vi "Process_Event.vi"(8 "Status/Errors in":refnum<vi>, 9 "Control Parameters [] in":T16[](array[typedef]) {"Aux Byte Value" format="%02x"; "Max Real Value" format="%#_6e"; "Min Real Value" format="%#_6e"; "dReal/dByte" format="%#_6e"; "Byte Value" format="%02x"; "Identifier" format="%02x"}, 10 "Main parameters in":T1={"Mode"={"Mode"=enum."Dialog", "Expert?"=FALSE, "Dialog?"=FALSE}, "Stop loop"={"Settings changed?"=FALSE, "Stop?"=refnum}, "Send message"={"Send mode"=enum."Get parameters", "Set parameter list"=0, "Get parameter list"=0, "Reset device"=0, "Length set settings message"=0, "Reset buttons?"=FALSE, "Reset Master?"=enum."General"}, "Write settings"={"Options"=enum."File 1"}, "Settings state"={"MAS locked?"=refnum, "SLV locked?"=refnum}, "Button refs"={"Stop program"=refnum, "Save settings"=refnum, "DAQ mode"=refnum, "Reset settings"=refnum, "Apply settings"=refnum, "Reset MAS"=refnum, "Reset SLV"=refnum, "Local DBase?"=refnum, "Last value DBase"=FALSE, "Database"=refnum, "Calibration"=refnum, "Save settings 2"=refnum}, "Update screen"={"Detector number"=0, "Hardware"=enum."None"}, "Files"={"Path config file"=path "", "Path def. ini file"=path "", "Path ini file 1"=path "", "Path ini file 2"=path "", "Path RBF file"=path ""}, "DB connection"={"connection reference"=refnum, "Connected?"=refnum, "ODBC Name"=""}, "Status_id"=refnum, "Time difference"=refnum, "Satellites"=refnum, "Alignment parameters"=refnum, "Page Statistics 2"=refnum, "Database"=refnum, "Page Statistics"=refnum} {"Update screen"."Detector number" format="%#.0f"; "Send message"."Reset device" format="%x"; "Send message"."Get parameter list" format="%x"; "Send message"."Set parameter list" format="%x"}, 11 "Event array":u8[](array[numeric])) -> (0 "Status/Errors out":refnum<vi>, 1 "Main parameters out":T1={"Mode"={"Mode"=enum."Dialog", "Expert?"=FALSE, "Dialog?"=FALSE}, "Stop loop"={"Settings changed?"=FALSE, "Stop?"=refnum}, "Send message"={"Send mode"=enum."Get parameters", "Set parameter list"=0, "Get parameter list"=0, "Reset device"=0, "Length set settings message"=0, "Reset buttons?"=FALSE, "Reset Master?"=enum."General"}, "Write settings"={"Options"=enum."File 1"}, "Settings state"={"MAS locked?"=refnum, "SLV locked?"=refnum}, "Button refs"={"Stop program"=refnum, "Save settings"=refnum, "DAQ mode"=refnum, "Reset settings"=refnum, "Apply settings"=refnum, "Reset MAS"=refnum, "Reset SLV"=refnum, "Local DBase?"=refnum, "Last value DBase"=FALSE, "Database"=refnum, "Calibration"=refnum, "Save settings 2"=refnum}, "Update screen"={"Detector number"=0, "Hardware"=enum."None"}, "Files"={"Path config file"=path "", "Path def. ini file"=path "", "Path ini file 1"=path "", "Path ini file 2"=path "", "Path RBF file"=path ""}, "DB connection"={"connection reference"=refnum, "Connected?"=refnum, "ODBC Name"=""}, "Status_id"=refnum, "Time difference"=refnum, "Satellites"=refnum, "Alignment parameters"=refnum, "Page Statistics 2"=refnum, "Database"=refnum, "Page Statistics"=refnum} {"Update screen"."Detector number" format="%#.0f"; "Send message"."Reset device" format="%x"; "Send message"."Get parameter list" format="%x"; "Send message"."Set parameter list" format="%x"}, 2 "Event statistics":T15[](array[typedef]), 3 "Event cluster":T17={"Det_Numb"=0, "GPS_Timestamp"="", "Trigger_Pattern"={"Master ch. 1 lower threshold"=FALSE, "Master ch. 1 higher threshold"=FALSE, "Master ch. 2 lower threshold"=FALSE, "Master ch. 2 higher threshold"=FALSE, "Slave ch. 1 lower threshold"=FALSE, "Slave ch. 1 higher threshold"=FALSE, "Slave ch. 2 lower threshold"=FALSE, "Slave ch. 2 higher threshold"=FALSE, "External trigger"=FALSE, "Slave present?"=FALSE, "Ch. 1 low comparator master"=FALSE, "Ch. 1 high comparator master"=FALSE, "Ch. 2 low comparator master"=FALSE, "Ch. 2 high comparator master"=FALSE, "Ch. 1 low comparator slave"=FALSE, "Ch. 1 high comparator slave"=FALSE, "Ch. 2 low comparator slave"=FALSE, "Ch. 2 high comparator slave"=FALSE}, "Traces"=[], "MAS_Status_Events"=FALSE, "MAS_Vers_Numb"="Hardware: 0    FPGA: 0", "SLV_Status_Events"=FALSE, "SLV_Vers_Numb"="Hardware: 0    FPGA: 0", "DBase_connected?"=FALSE, "MAS_GPS_Long"=0.0, "MAS_GPS_Lat"=0.0, "MAS_GPS_Alt"=0.0, "Hardware"=enum."None"} {"MAS_GPS_Alt" format="%.2g"; "MAS_GPS_Lat" format="%#.7f"; "MAS_GPS_Long" format="%#.7f"})   [LabVIEW 2013]
uses:
  Controls/TabPage_Events.ctl
  Controls/Control_Parameters.ctl
  Controls/Master.ctl
  Controls/Event_Statistics.ctl
  Controls/Main_Parameters.ctl
  Controls/Mode.ctl
  Controls/Stop_Loop.ctl
  Controls/Send_Message.ctl
  Controls/Send_Message_Mode.ctl
  Controls/Write_Settings.ctl
  Controls/Write_Settings_Options.ctl
  Controls/Settings_State.ctl
  Controls/Button_Refs.ctl
  Controls/Update_Screen.ctl
  Controls/Files.ctl
  Controls/DB_Connection.ctl
  database/Connection.llb/Conn ObjectReference.ctl
  Controls/Get_Set_Statistics_Options2.ctl
panel:
  in  "Start counting?":bool=TRUE
  out "timer":u32
  in  "Start counting":bool=TRUE
  out "timer":u32
  out "Last trace":dbl[][](array[numeric])
  out "Show traces? 2":bool
  out "Show traces?":bool
  out "Last trace":dbl[][](array[numeric])
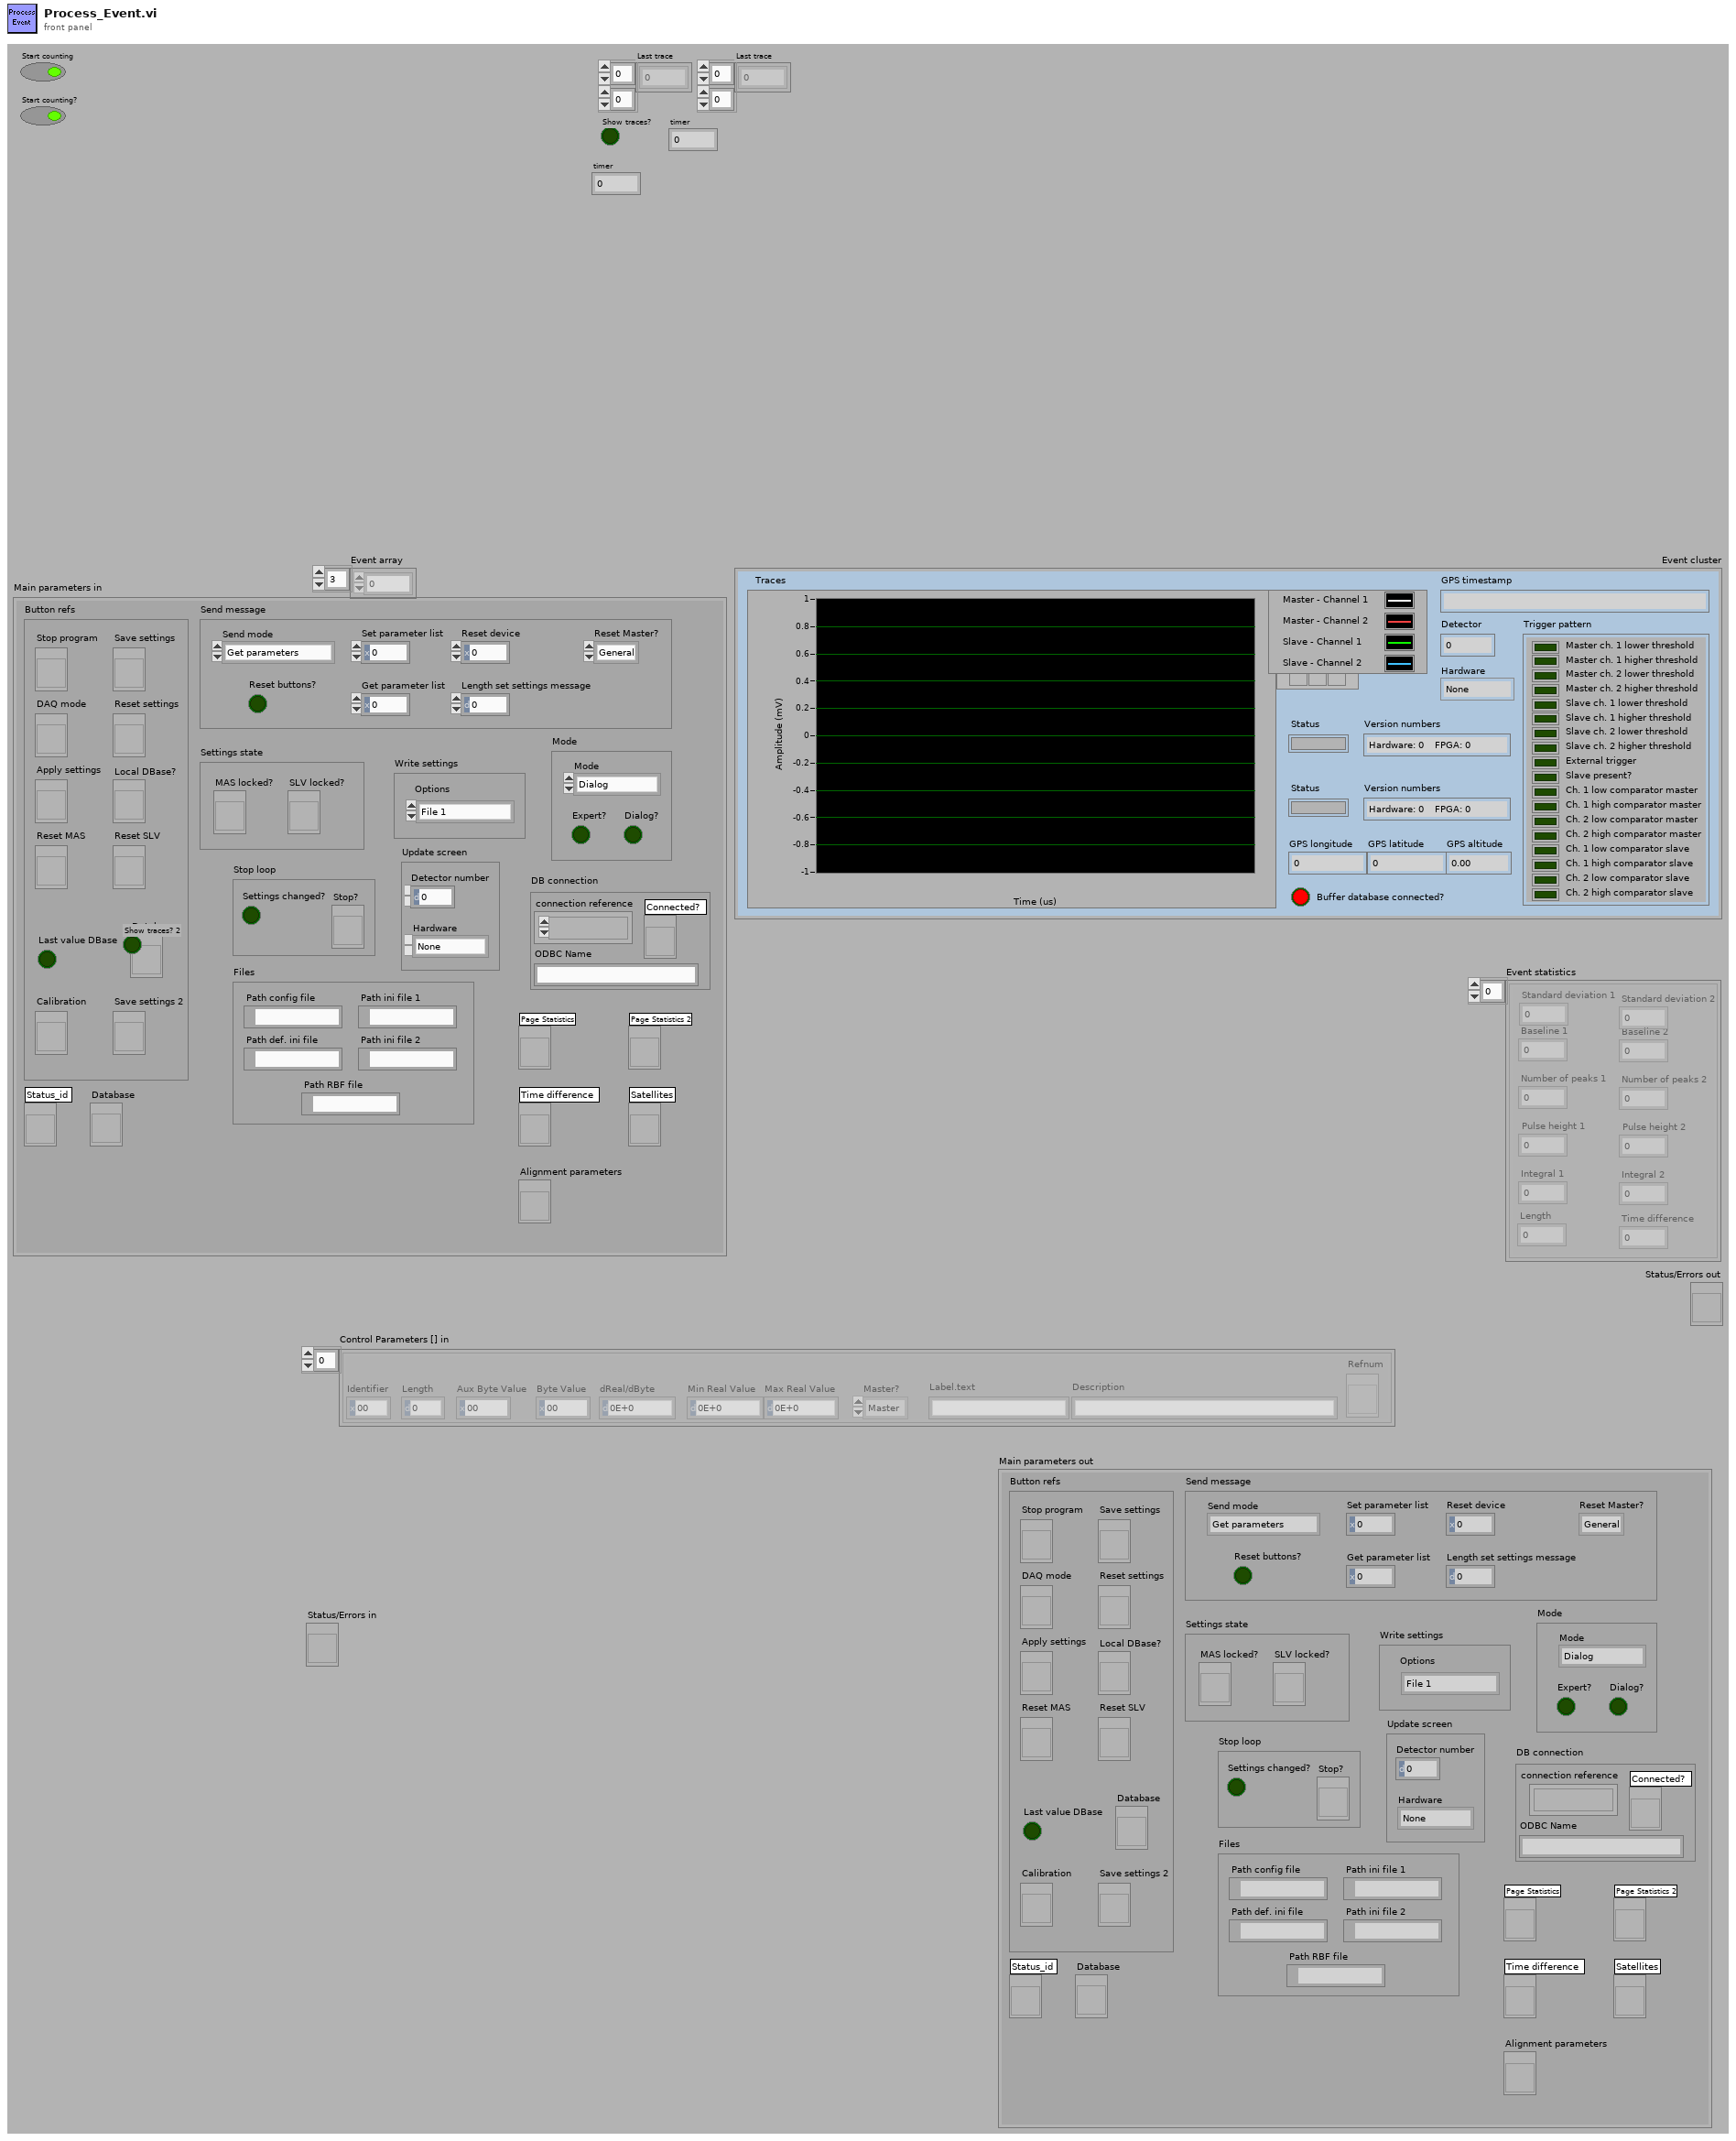
[diagram p1: front panel]
types:
  T1 = typedef "Main_Parameters.ctl" = cluster{"Mode":T2, "Stop loop":T3, "Send message":T4, "Write settings":T7, "Settings state":T9, "Button refs":T10, "Update screen":T11, "Files":T12, "DB connection":T13, "Status_id":refnum<vi>, "Time difference":refnum<vi>, "Satellites":refnum<vi>, "Alignment parameters":refnum<vi>, "Page Statistics 2":refnum<vi>, "Database":refnum<vi>, "Page Statistics":refnum<vi>}
  T2 = typedef "Mode.ctl" = cluster{"Mode":enum8{"Stop", "Dialog", "Hisparc II", "Hisparc II DAQ", "Alignment"}, "Expert?":bool, "Dialog?":bool}
  T3 = typedef "Stop_Loop.ctl" = cluster{"Settings changed?":bool, "Stop?":refnum<vi>}
  T4 = typedef "Send_Message.ctl" = cluster{"Send mode":T5, "Set parameter list":u8, "Get parameter list":u8, "Reset device":u8, "Length set settings message":i32, "Reset buttons?":bool, "Reset Master?":T6}
  T5 = typedef "Send_Message_Mode.ctl" = enum16{"Get parameters", "Set parameters", "From front panel", "From parameters", "Reset device", "Alignment"}
  T6 = typedef "Master.ctl" = enum16{"Master", "Slave", "General"}
  T7 = typedef "Write_Settings.ctl" = cluster{"Options":T8}
  T8 = typedef "Write_Settings_Options.ctl" = enum16{"File 1", "File 2", "Alignment", "Reset"}
  T9 = typedef "Settings_State.ctl" = cluster{"MAS locked?":refnum<vi>, "SLV locked?":refnum<vi>}
  T10 = typedef "Button_Refs.ctl" = cluster{"Stop program":refnum<vi>, "Save settings":refnum<vi>, "DAQ mode":refnum<vi>, "Reset settings":refnum<vi>, "Apply settings":refnum<vi>, "Reset MAS":refnum<vi>, "Reset SLV":refnum<vi>, "Local DBase?":refnum<vi>, "Last value DBase":bool, "Database":refnum<vi>, "Calibration":refnum<vi>, "Save settings 2":refnum<vi>}
  T11 = typedef "Update_Screen.ctl" = cluster{"Detector number":u16, "Hardware":enum8{"None", "HiSPARC I", "HiSPARC II", "HiSPARC III", "Unknown"}}
  T12 = typedef "Files.ctl" = cluster{"Path config file":path, "Path def. ini file":path, "Path ini file 1":path, "Path ini file 2":path, "Path RBF file":path}
  T13 = typedef "DB_Connection.ctl" = cluster{"connection reference":T14, "Connected?":refnum<vi>, "ODBC Name":string}
  T14 = typedef "Conn ObjectReference.ctl" = refnum<k1>
  T15 = typedef "Event_Statistics.ctl" = cluster{"Baseline 1":i16, "Baseline 2":i16, "Number of peaks 1":i16, "Number of peaks 2":i16, "Pulse height 1":i16, "Pulse height 2":i16, "Integral 1":i32, "Integral 2":i32, "Standard deviation 1":i16, "Standard deviation 2":i16, "Length":i32, "Time difference":u32}
  T16 = typedef "Control_Parameters.ctl" = cluster{"Identifier":u8, "Length":u16, "Byte Value":u32, "dReal/dByte":dbl, "Min Real Value":dbl, "Max Real Value":dbl, "Master?":T6, "Label.text":string, "Description":string, "Refnum":refnum<vi>, "Aux Byte Value":u32}
  T17 = typedef "TabPage_Events.ctl" = cluster{"Det_Numb":u16, "GPS_Timestamp":string, "Trigger_Pattern":cluster{"Master ch. 1 lower threshold":bool, "Master ch. 1 higher threshold":bool, "Master ch. 2 lower threshold":bool, "Master ch. 2 higher threshold":bool, "Slave ch. 1 lower threshold":bool, "Slave ch. 1 higher threshold":bool, "Slave ch. 2 lower threshold":bool, "Slave ch. 2 higher threshold":bool, "External trigger":bool, "Slave present?":bool, "Ch. 1 low comparator master":bool, "Ch. 1 high comparator master":bool, "Ch. 2 low comparator master":bool, "Ch. 2 high comparator master":bool, "Ch. 1 low comparator slave":bool, "Ch. 1 high comparator slave":bool, "Ch. 2 low comparator slave":bool, "Ch. 2 high comparator slave":bool}, "Traces":dbl[][], "MAS_Status_Events":bool, "MAS_Vers_Numb":string, "SLV_Status_Events":bool, "SLV_Vers_Numb":string, "DBase_connected?":bool, "MAS_GPS_Long":dbl, "MAS_GPS_Lat":dbl, "MAS_GPS_Alt":dbl, "Hardware":enum8{"None", "HiSPARC I", "HiSPARC II", "HiSPARC III", "Unknown"}}
  T18 = typedef "Get_Set_Statistics_Options2.ctl" = enum16{"Get", "Set"}
  T19 = enum8{"None", "HiSPARC I", "HiSPARC II", "HiSPARC III", "Unknown"}
  T20 = cluster{"Last trigger":u64, "Time difference":u64}
  T21 = cluster{"dReal/dByte":dbl, "dReal/dByte":dbl, "dReal/dByte":dbl, "dReal/dByte 2":dbl}
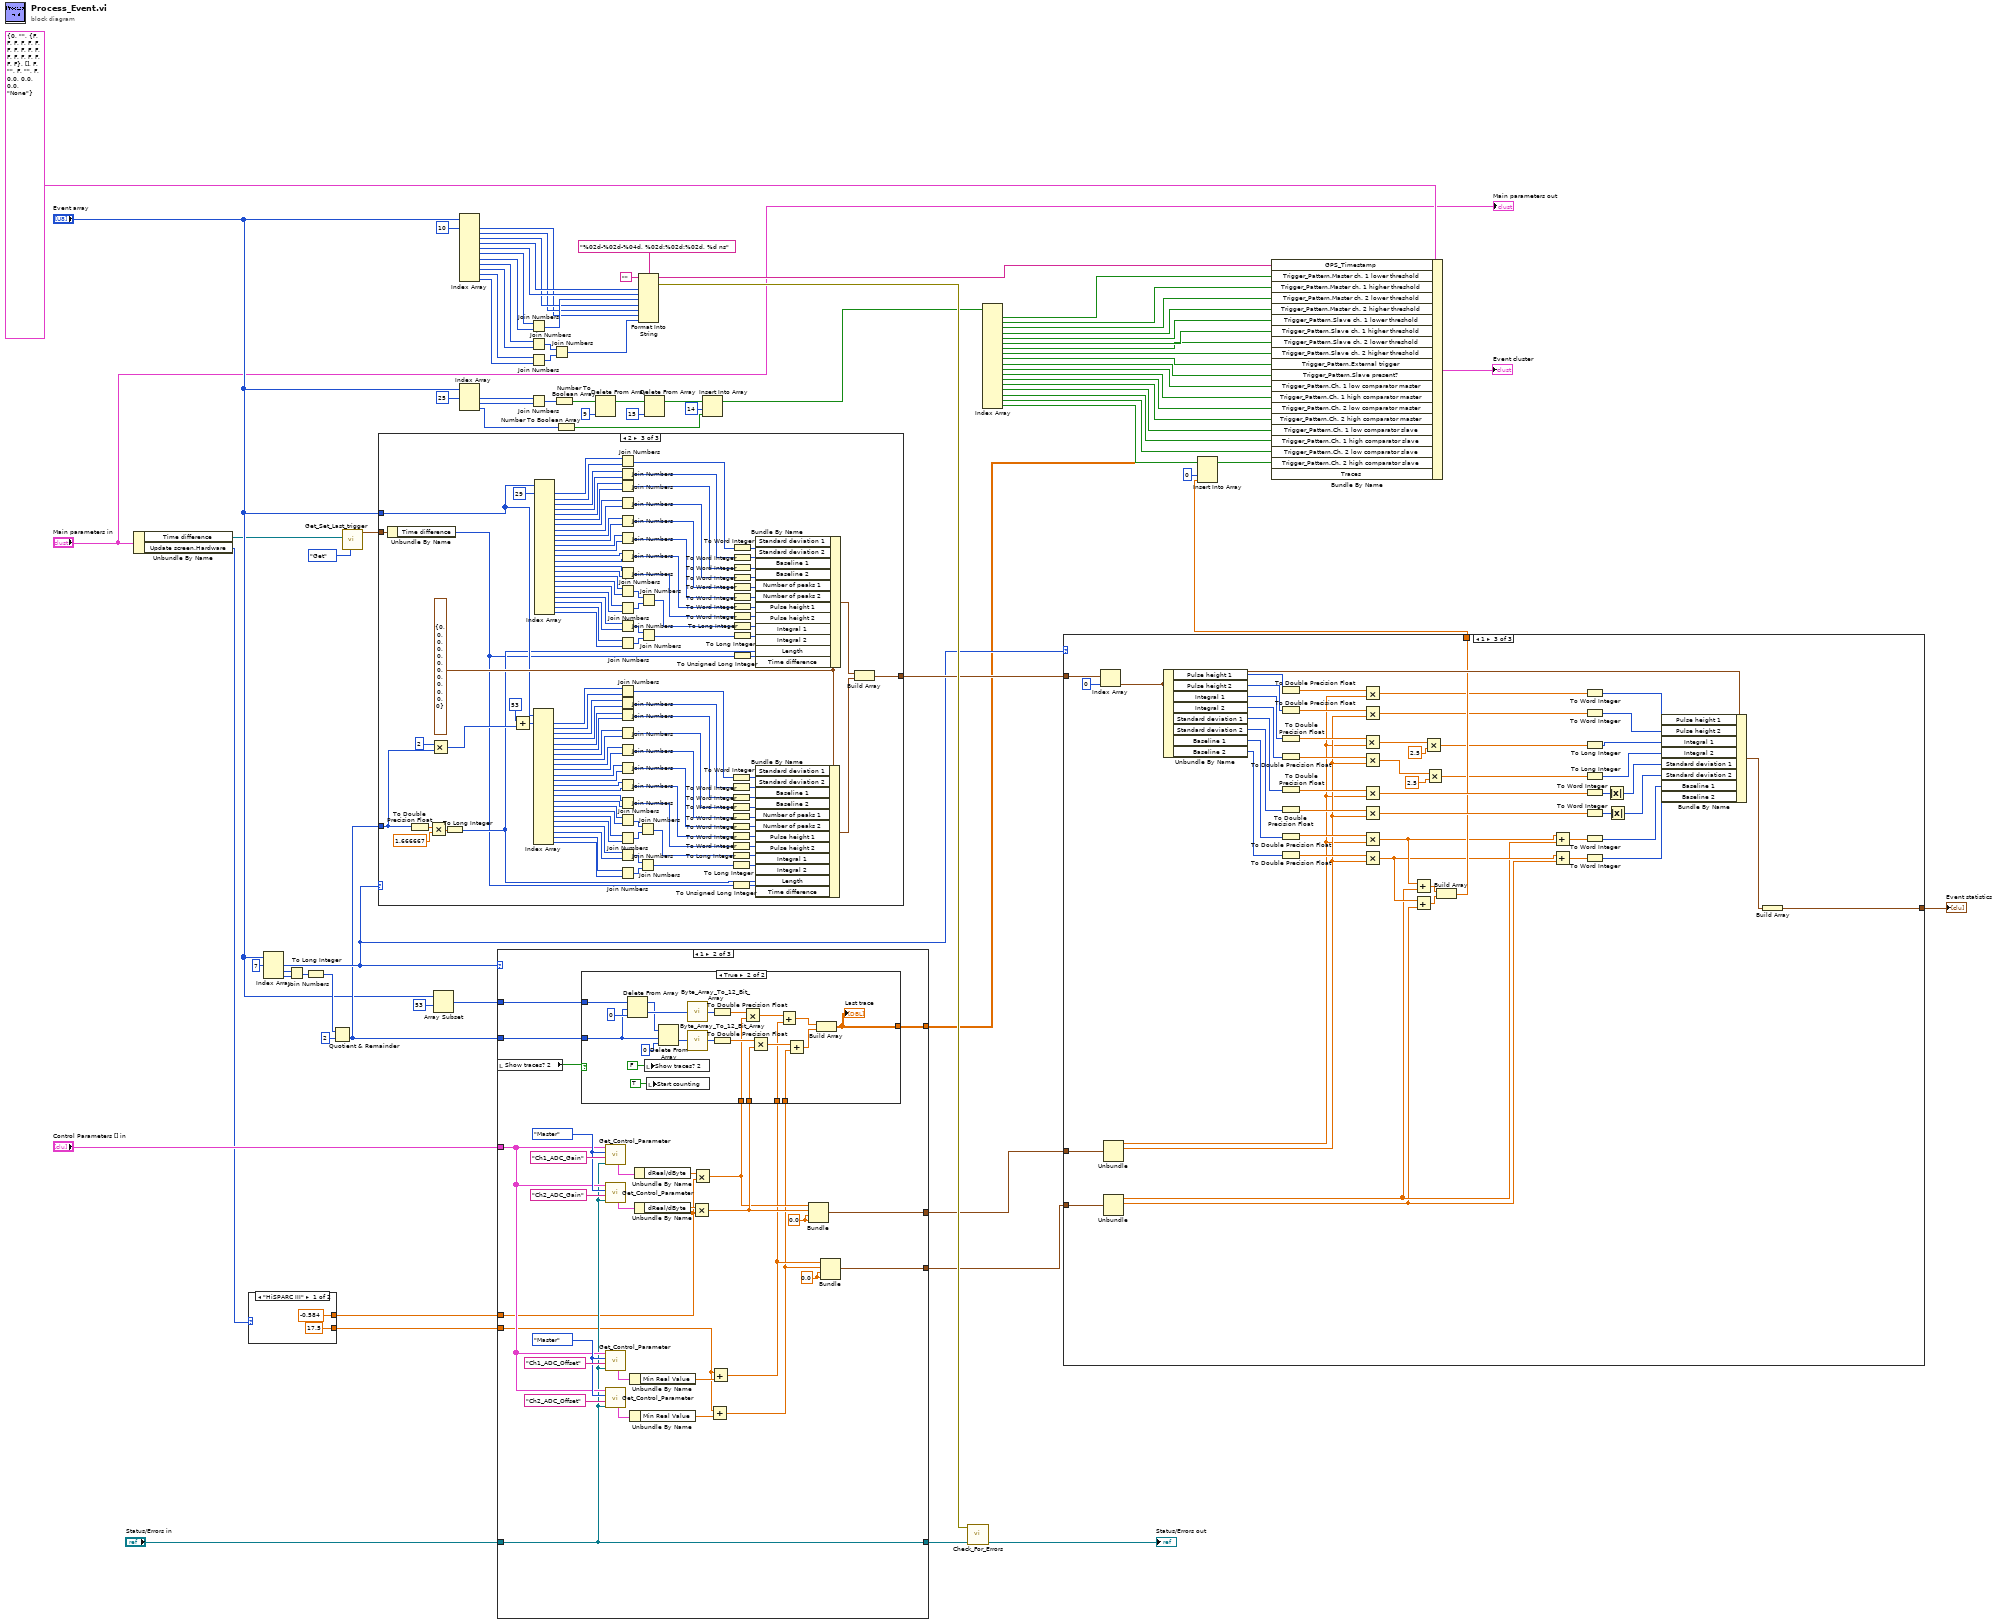
[diagram p0: block diagram]
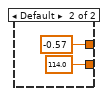
[diagram p2: hidden frame]
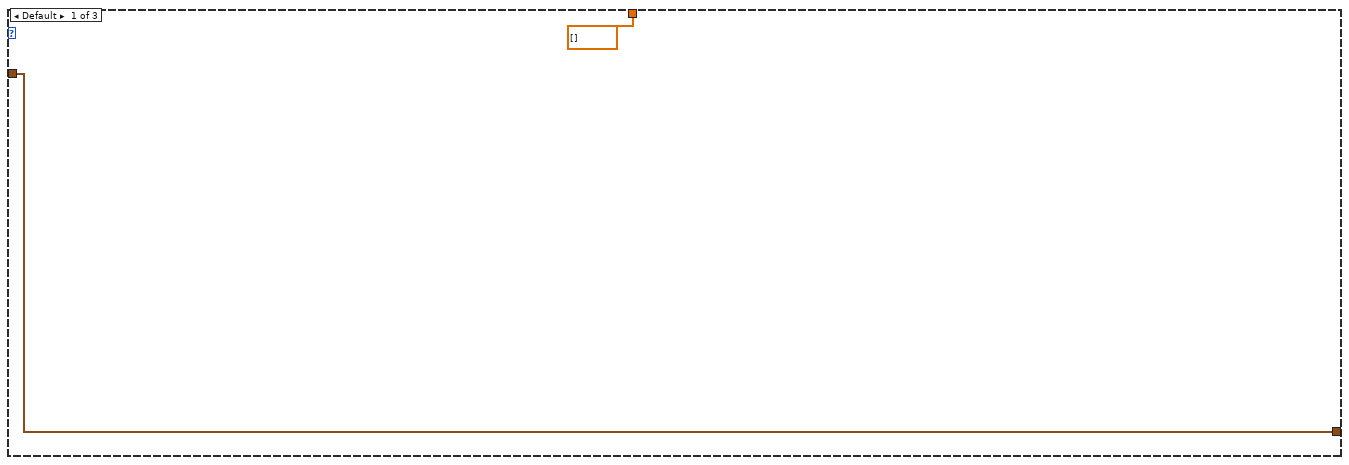
[diagram p3: hidden frame]
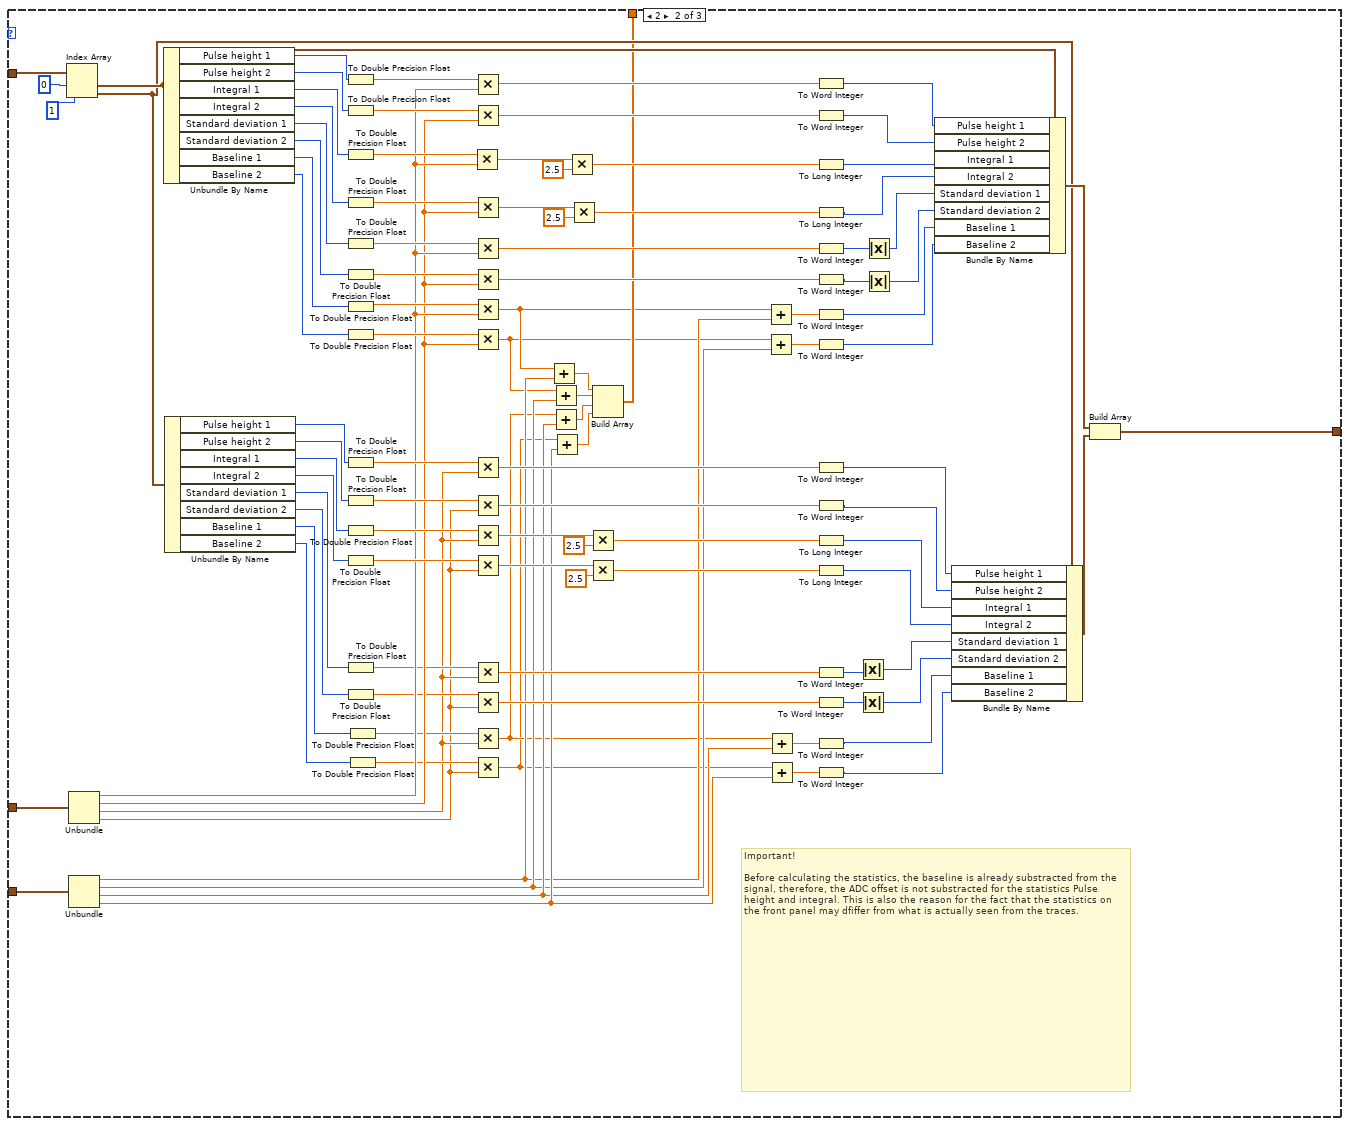
[diagram p4: hidden frame]
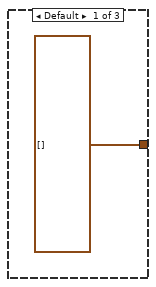
[diagram p5: hidden frame]
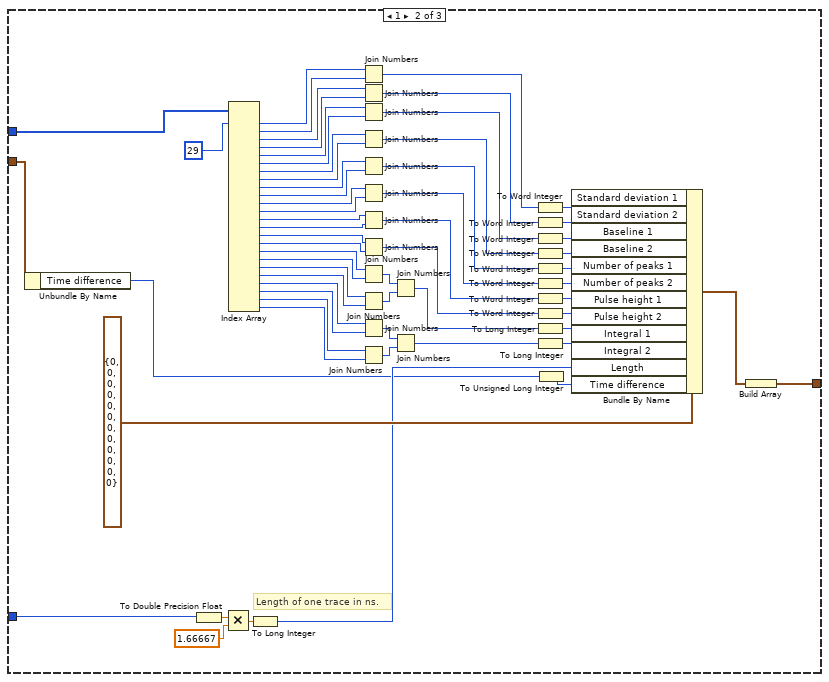
[diagram p6: hidden frame]
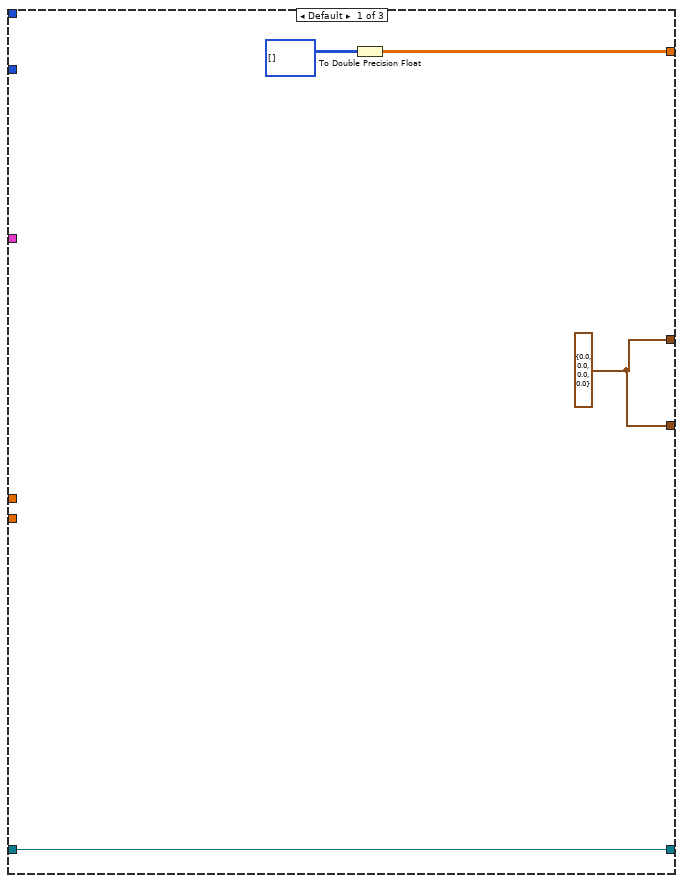
[diagram p7: hidden frame]
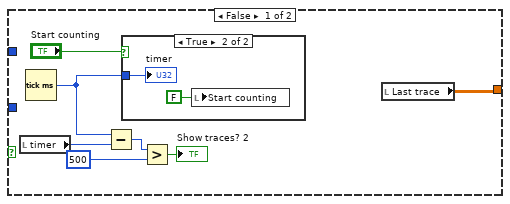
[diagram p8: hidden frame]
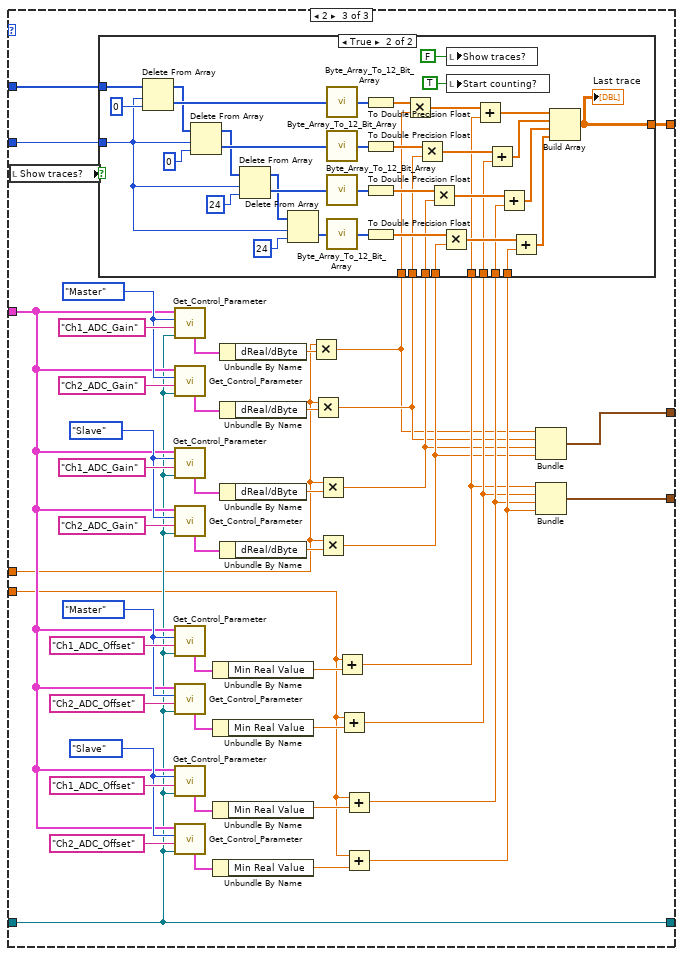
[diagram p10: hidden frame]
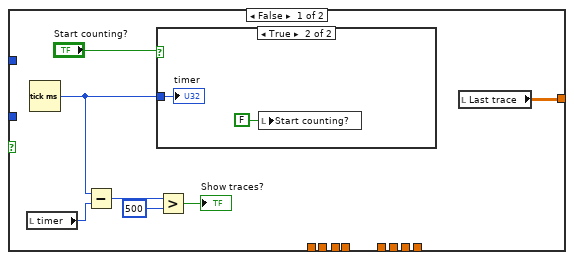
[diagram p11: hidden frame]
diagram:
  n1 = Unbundle By Name("Main parameters in") -> ("Time difference"=w34:refnum<vi>, "Update screen.Hardware"=w3:T19)
  n2 = case shown="\"HiSPARC III\"" w3 {
    tunnel: [-0.584 ("y") -0.57 ("y")] -> w2
    tunnel: [17.5 ("x") 114.0 ("x")] -> w1
    frame "HiSPARC III" {
    }
    frame Default {
    }
  }
  n3 = Index Array(array="Event array", index #1=7 ("index")) -> (element #1=w40:u8, element #2=w55:u8, element #3=w54:u8)  [unwired: 2 in]
  n4 = Join Numbers(hi=w55, lo=w54) -> ((hi.lo)=w44:u16)
  n5 = To Long Integer(number=w44) -> (32bit integer=w38:i32)
  n6 = Quotient & Remainder(x=w38, y=2) -> (floor(x/y)=w37:i32)  [unwired: 1 out]
  n7 = call "Get_Set_Last_trigger.vi"("Get/Set"=Get_Set_Statistics_Options2."Get", "Time difference"=w34) -> ("Value out"=w32:T20)  [unwired: 2 in, 7 out]
  n8 = case shown="2" w40 {
    tunnel: "Event array" -> [_ w101 w162]
    tunnel: [T15[] [] w98 w224] -> w43
    tunnel: w37 -> [_ w93 w155]
    tunnel: w32 -> [_ w91 w153]
    frame Default {
    }
    frame 1 {
      # "Length of one trace in ns."
      n9 = Unbundle By Name(w91) -> ("Time difference"=w90:u64)
      n10 = To Double Precision Float(number=w93) -> (double precision float=w95:dbl)
      n11 = Multiply(x=w95, y=1.66667) -> (x*y=w94:dbl)
      n12 = Index Array(array=w101, index #1=29 ("index")) -> (element #1=w110:u8, element #2=w109:u8, element #3=w107:u8, element #4=w108:u8, element #5=w149:u8, element #6=w148:u8, element #7=w145:u8, element #8=w144:u8, element #9=w143:u8, element #10=w142:u8, element #11=w141:u8, element #12=w140:u8, element #13=w139:u8, element #14=w138:u8, element #15=w137:u8, element #16=w136:u8, element #17=w135:u8, element #18=w134:u8, element #19=w133:u8, element #20=w132:u8, element #21=w129:u8, element #22=w128:u8, element #23=w127:u8, element #24=w126:u8)  [unwired: 23 in]
      n13 = To Long Integer(number=w94) -> (32bit integer=w92:i32)
      n14 = Join Numbers(hi=w110, lo=w109) -> ((hi.lo)=w106:u16)
      n15 = Join Numbers(hi=w107, lo=w108) -> ((hi.lo)=w103:u16)
      n16 = Join Numbers(hi=w149, lo=w148) -> ((hi.lo)=w125:u16)
      n17 = Join Numbers(hi=w145, lo=w144) -> ((hi.lo)=w117:u16)
      n18 = Join Numbers(hi=w143, lo=w142) -> ((hi.lo)=w116:u16)
      n19 = Join Numbers(hi=w141, lo=w140) -> ((hi.lo)=w115:u16)
      n20 = Join Numbers(hi=w139, lo=w138) -> ((hi.lo)=w114:u16)
      n21 = Join Numbers(hi=w137, lo=w136) -> ((hi.lo)=w113:u16)
      n22 = Join Numbers(hi=w135, lo=w134) -> ((hi.lo)=w147:u16)
      n23 = Join Numbers(hi=w133, lo=w132) -> ((hi.lo)=w146:u16)
      n24 = Join Numbers(hi=w129, lo=w128) -> ((hi.lo)=w131:u16)
      n25 = Join Numbers(hi=w127, lo=w126) -> ((hi.lo)=w130:u16)
      n26 = Join Numbers(hi=w147, lo=w146) -> ((hi.lo)=w112:u32)
      n27 = Join Numbers(hi=w131, lo=w130) -> ((hi.lo)=w111:u32)
      n28 = To Word Integer(number=w106) -> (16bit integer=w105:i16)
      n29 = To Word Integer(number=w103) -> (16bit integer=w104:i16)
      n30 = To Word Integer(number=w125) -> (16bit integer=w124:i16)
      n31 = To Word Integer(number=w117) -> (16bit integer=w123:i16)
      n32 = To Word Integer(number=w116) -> (16bit integer=w122:i16)
      n33 = To Word Integer(number=w115) -> (16bit integer=w121:i16)
      n34 = To Word Integer(number=w114) -> (16bit integer=w120:i16)
      n35 = To Word Integer(number=w113) -> (16bit integer=w119:i16)
      n36 = To Long Integer(number=w112) -> (32bit integer=w89:i32)
      n37 = To Long Integer(number=w111) -> (32bit integer=w118:i32)
      n38 = To Unsigned Long Integer(number=w90) -> (unsigned 32bit integer=w97:u32)
      n39 = Bundle By Name(cluster=T15 {"Baseline 1"=0, "Baseline 2"=0, "Number of peaks 1"=0, "Number of peaks 2"=0, "Pulse height 1"=0, "Pulse height 2"=0, "Integral 1"=0, "Integral 2"=0, "Standard deviation 1"=0, "Standard deviation 2"=0, "Length"=0, "Time difference"=0} ("Event statistics"), "Standard deviation 1"=w105, "Standard deviation 2"=w104, "Baseline 1"=w124, "Baseline 2"=w123, "Number of peaks 1"=w122, "Number of peaks 2"=w121, "Pulse height 1"=w120, "Pulse height 2"=w119, "Integral 1"=w89, "Integral 2"=w118, "Length"=w92, "Time difference"=w97) -> (w102:T15)
      n40 = Build Array(w102) -> (w98:T15[])
    }
    frame 2 {
      w167 = T15 {"Baseline 1"=0, "Baseline 2"=0, "Number of peaks 1"=0, "Number of peaks 2"=0, "Pulse height 1"=0, "Pulse height 2"=0, "Integral 1"=0, "Integral 2"=0, "Standard deviation 1"=0, "Standard deviation 2"=0, "Length"=0, "Time difference"=0} ("Event statistics")
      n41 = Unbundle By Name(w153) -> ("Time difference"=w151:u64)
      n42 = To Double Precision Float(number=w155) -> (double precision float=w158:dbl)
      n43 = Multiply(x=w158, y=1.666667) -> (x*y=w157:dbl)
      n44 = Multiply(x=2, y=w155) -> (x*y=w156:i32)
      n45 = To Long Integer(number=w157) -> (32bit integer=w152:i32)
      n46 = Add(x=53 ("index"), y=w156) -> (x+y=w163:i32)
      n47 = Index Array(array=w162, index #1=w163) -> (element #1=w165:u8, element #2=w164:u8, element #3=w173:u8, element #4=w174:u8, element #5=w214:u8, element #6=w213:u8, element #7=w210:u8, element #8=w209:u8, element #9=w208:u8, element #10=w207:u8, element #11=w206:u8, element #12=w205:u8, element #13=w204:u8, element #14=w203:u8, element #15=w202:u8, element #16=w201:u8, element #17=w200:u8, element #18=w199:u8, element #19=w198:u8, element #20=w197:u8, element #21=w194:u8, element #22=w193:u8, element #23=w192:u8, element #24=w191:u8)  [unwired: 23 in]
      n48 = Index Array(array=w162, index #1=29 ("index")) -> (element #1=w222:u8, element #2=w221:u8, element #3=w219:u8, element #4=w220:u8, element #5=w264:u8, element #6=w263:u8, element #7=w260:u8, element #8=w259:u8, element #9=w258:u8, element #10=w257:u8, element #11=w256:u8, element #12=w255:u8, element #13=w254:u8, element #14=w253:u8, element #15=w252:u8, element #16=w251:u8, element #17=w250:u8, element #18=w249:u8, element #19=w248:u8, element #20=w247:u8, element #21=w244:u8, element #22=w243:u8, element #23=w242:u8, element #24=w241:u8)  [unwired: 23 in]
      n49 = Join Numbers(hi=w165, lo=w164) -> ((hi.lo)=w172:u16)
      n50 = Join Numbers(hi=w173, lo=w174) -> ((hi.lo)=w169:u16)
      n51 = Join Numbers(hi=w214, lo=w213) -> ((hi.lo)=w190:u16)
      n52 = Join Numbers(hi=w210, lo=w209) -> ((hi.lo)=w181:u16)
      n53 = Join Numbers(hi=w208, lo=w207) -> ((hi.lo)=w180:u16)
      n54 = Join Numbers(hi=w206, lo=w205) -> ((hi.lo)=w179:u16)
      n55 = Join Numbers(hi=w204, lo=w203) -> ((hi.lo)=w178:u16)
      n56 = Join Numbers(hi=w202, lo=w201) -> ((hi.lo)=w177:u16)
      n57 = Join Numbers(hi=w200, lo=w199) -> ((hi.lo)=w212:u16)
      n58 = Join Numbers(hi=w198, lo=w197) -> ((hi.lo)=w211:u16)
      n59 = Join Numbers(hi=w194, lo=w193) -> ((hi.lo)=w196:u16)
      n60 = Join Numbers(hi=w192, lo=w191) -> ((hi.lo)=w195:u16)
      n61 = Join Numbers(hi=w222, lo=w221) -> ((hi.lo)=w218:u16)
      n62 = Join Numbers(hi=w219, lo=w220) -> ((hi.lo)=w215:u16)
      n63 = Join Numbers(hi=w264, lo=w263) -> ((hi.lo)=w240:u16)
      n64 = Join Numbers(hi=w260, lo=w259) -> ((hi.lo)=w232:u16)
      n65 = Join Numbers(hi=w258, lo=w257) -> ((hi.lo)=w231:u16)
      n66 = Join Numbers(hi=w256, lo=w255) -> ((hi.lo)=w230:u16)
      n67 = Join Numbers(hi=w254, lo=w253) -> ((hi.lo)=w229:u16)
      n68 = Join Numbers(hi=w252, lo=w251) -> ((hi.lo)=w228:u16)
      n69 = Join Numbers(hi=w250, lo=w249) -> ((hi.lo)=w262:u16)
      n70 = Join Numbers(hi=w248, lo=w247) -> ((hi.lo)=w261:u16)
      n71 = Join Numbers(hi=w244, lo=w243) -> ((hi.lo)=w246:u16)
      n72 = Join Numbers(hi=w242, lo=w241) -> ((hi.lo)=w245:u16)
      n73 = Join Numbers(hi=w212, lo=w211) -> ((hi.lo)=w176:u32)
      n74 = Join Numbers(hi=w196, lo=w195) -> ((hi.lo)=w175:u32)
      n75 = Join Numbers(hi=w262, lo=w261) -> ((hi.lo)=w227:u32)
      n76 = Join Numbers(hi=w246, lo=w245) -> ((hi.lo)=w226:u32)
      n77 = To Word Integer(number=w172) -> (16bit integer=w171:i16)
      n78 = To Word Integer(number=w169) -> (16bit integer=w170:i16)
      n79 = To Word Integer(number=w190) -> (16bit integer=w189:i16)
      n80 = To Word Integer(number=w181) -> (16bit integer=w188:i16)
      n81 = To Word Integer(number=w180) -> (16bit integer=w187:i16)
      n82 = To Word Integer(number=w179) -> (16bit integer=w186:i16)
      n83 = To Word Integer(number=w178) -> (16bit integer=w185:i16)
      n84 = To Word Integer(number=w177) -> (16bit integer=w184:i16)
      n85 = To Long Integer(number=w176) -> (32bit integer=w183:i32)
      n86 = To Long Integer(number=w175) -> (32bit integer=w182:i32)
      n87 = To Unsigned Long Integer(number=w151) -> (unsigned 32bit integer=w160:u32)
      n88 = To Word Integer(number=w218) -> (16bit integer=w217:i16)
      n89 = To Word Integer(number=w215) -> (16bit integer=w216:i16)
      n90 = To Word Integer(number=w240) -> (16bit integer=w239:i16)
      n91 = To Word Integer(number=w232) -> (16bit integer=w238:i16)
      n92 = To Word Integer(number=w231) -> (16bit integer=w237:i16)
      n93 = To Word Integer(number=w230) -> (16bit integer=w236:i16)
      n94 = To Word Integer(number=w229) -> (16bit integer=w235:i16)
      n95 = To Word Integer(number=w228) -> (16bit integer=w234:i16)
      n96 = To Long Integer(number=w227) -> (32bit integer=w150:i32)
      n97 = To Long Integer(number=w226) -> (32bit integer=w233:i32)
      n98 = To Unsigned Long Integer(number=w151) -> (unsigned 32bit integer=w161:u32)
      n99 = Bundle By Name(cluster=w167, "Standard deviation 1"=w171, "Standard deviation 2"=w170, "Baseline 1"=w189, "Baseline 2"=w188, "Number of peaks 1"=w187, "Number of peaks 2"=w186, "Pulse height 1"=w185, "Pulse height 2"=w184, "Integral 1"=w183, "Integral 2"=w182, "Length"=w152, "Time difference"=w160) -> (w168:T15)
      n100 = Bundle By Name(cluster=w167, "Standard deviation 1"=w217, "Standard deviation 2"=w216, "Baseline 1"=w239, "Baseline 2"=w238, "Number of peaks 1"=w237, "Number of peaks 2"=w236, "Pulse height 1"=w235, "Pulse height 2"=w234, "Integral 1"=w150, "Integral 2"=w233, "Length"=w152, "Time difference"=w161) -> (w225:T15)
      n101 = Build Array(w225, w168) -> (w224:T15[])
    }
  }
  n102 = Array Subset(array="Event array", index=53) -> (w46:u8[])  [unwired: 1 in]
  n103 = Index Array(array="Event array", index #1=10 ("index")) -> (element #1=w66:u8, element #2=w67:u8, element #3=w68:u8, element #4=w71:u8, element #5=w70:u8, element #6=w81:u8, element #7=w82:u8, element #8=w78:u8, element #9=w77:u8, element #10=w76:u8, element #11=w75:u8)  [unwired: 10 in]
  n104 = Index Array(array="Event array", index #1=25 ("index")) -> (element #1=w63:u8, element #2=w62:u8, element #3=w30:u8)  [unwired: 2 in]
  n105 = case shown="1" w40 {
    tunnel: w37 -> [_ w284 w351]
    tunnel: [w267 w298 w375] -> w6
    tunnel: w46 -> [_ w285 w352]
    tunnel: "Control Parameters [] in" -> [_ w287 w354]
    tunnel: "Status/Errors in" -> [w266 w286 w353]
    tunnel: [w266 w286 w353] -> w47
    tunnel: [w265 w283 w350] -> w39
    tunnel: [w265 w280 w349] -> w36
    tunnel: w2 -> [_ w269 w331]
    tunnel: w1 -> [_ w270 w330]
    frame Default {
      w265 = T21 {"dReal/dByte"=0.0, "dReal/dByte"=0.0, "dReal/dByte"=0.0, "dReal/dByte 2"=0.0}
      n106 = To Double Precision Float(number=u16[][] []) -> (double precision float=w267:dbl[][])
    }
    frame 1 {
      w281 = 0.0
      w282 = 0.0
      w288 = Master."Master" ("Master?")
      w293 = Master."Master" ("Master?")
      n107 = local read "Show traces? 2"() -> (w271:bool)
      n108 = call "Get_Control_Parameter.vi"("Status/Errors in"=w286, "Label.text in"="Ch1_ADC_Gain", "Master?"=w293, "Control Parameters [] in"=w287) -> ("Control Parameter"=w296:T16)  [unwired: 7 out]
      n109 = call "Get_Control_Parameter.vi"("Status/Errors in"=w286, "Label.text in"="Ch2_ADC_Gain", "Master?"=w293, "Control Parameters [] in"=w287) -> ("Control Parameter"=w294:T16)  [unwired: 7 out]
      n110 = call "Get_Control_Parameter.vi"("Status/Errors in"=w286, "Label.text in"="Ch1_ADC_Offset", "Master?"=w288, "Control Parameters [] in"=w287) -> ("Control Parameter"=w291:T16)  [unwired: 7 out]
      n111 = call "Get_Control_Parameter.vi"("Status/Errors in"=w286, "Label.text in"="Ch2_ADC_Offset", "Master?"=w288, "Control Parameters [] in"=w287) -> ("Control Parameter"=w289:T16)  [unwired: 7 out]
      n112 = Unbundle By Name(w291) -> ("Min Real Value"=w275:dbl)
      n113 = Unbundle By Name(w289) -> ("Min Real Value"=w274:dbl)
      n114 = Unbundle By Name(w296) -> ("dReal/dByte"=w279:dbl)
      n115 = Unbundle By Name(w294) -> ("dReal/dByte"=w278:dbl)
      n116 = Multiply(x=w278, y=w269) -> (x*y=w277:dbl)
      n117 = Multiply(x=w279, y=w269) -> (x*y=w276:dbl)
      n118 = Add(x=w270, y=w274) -> (x+y=w272:dbl)
      n119 = Add(x=w270, y=w275) -> (x+y=w273:dbl)
      n120 = case shown="True" w271 {
        tunnel: [w303 w329] -> w298
        tunnel: w285 -> [_ w320]
        tunnel: w284 -> [_ w315]
        tunnel: w277 -> [_ w313]
        tunnel: w276 -> [_ w312]
        tunnel: w273 -> [_ w311]
        tunnel: w272 -> [_ w310]
        frame False {
          n121 = local read "timer"() -> (w300:u32)
          n122 = Tick Count (ms)() -> (millisecond timer value=w301:u32)
          n123 = Subtract(x=w301, y=w300) -> (x-y=w299:u32)
          n124 = case shown="True" "Start counting" {
            tunnel: w301 -> [_ w307]
            frame False {
            }
            frame True {
              n125 = local write "Start counting"(FALSE ("Start counting")) -> ()
              "timer" <- w307
            }
          }
          n126 = Greater?(x=w299, y=u32 500) -> (0:→"Show traces? 2":bool)
          n127 = local read "Last trace"() -> (w303:dbl[][])
        }
        frame True {
          n128 = Delete From Array(array=w320, length=w315, index=0) -> (deleted portion=w318:u8[], array with subset deleted=w316:u8[])
          n129 = local write "Show traces? 2"(FALSE ("Show traces? 2")) -> ()
          n130 = local write "Start counting"(TRUE ("Start counting")) -> ()
          n131 = Delete From Array(array=w316, length=w315, index=0) -> (deleted portion=w314:u8[])  [unwired: 1 out]
          n132 = call "Byte_Array_To_12_Bit_Array.vi"("Byte-Array"=w318) -> ("12-Bit-Array"=w328:u16[])
          n133 = call "Byte_Array_To_12_Bit_Array.vi"("Byte-Array"=w314) -> ("12-Bit-Array"=w322:u16[])
          n134 = To Double Precision Float(number=w328) -> (double precision float=w327:dbl[])
          n135 = To Double Precision Float(number=w322) -> (double precision float=w324:dbl[])
          n136 = Multiply(x=w327, y=w312) -> (x*y=w326:dbl[])
          n137 = Multiply(x=w324, y=w313) -> (x*y=w323:dbl[])
          n138 = Add(x=w326, y=w311) -> (x+y=w325:dbl[])
          n139 = Add(x=w323, y=w310) -> (x+y=w321:dbl[])
          n140 = Build Array(w325, w321) -> (w329:dbl[][])
          "Last trace" <- w329
        }
      }
      n141 = Bundle(w276, w277, w282, w282) -> (w283:cluster{dbl, dbl, dbl, dbl})  [unwired: 1 out]
      n142 = Bundle(w273, w272, w281, w281) -> (w280:cluster{dbl, dbl, dbl, dbl})  [unwired: 1 out]
    }
    frame 2 {
      w355 = Master."Slave" ("Master?")
      w360 = Master."Master" ("Master?")
      w365 = Master."Slave" ("Master?")
      w370 = Master."Master" ("Master?")
      n143 = local read "Show traces?"() -> (w332:bool)
      n144 = call "Get_Control_Parameter.vi"("Status/Errors in"=w353, "Label.text in"="Ch1_ADC_Gain", "Master?"=w370, "Control Parameters [] in"=w354) -> ("Control Parameter"=w373:T16)  [unwired: 7 out]
      n145 = call "Get_Control_Parameter.vi"("Status/Errors in"=w353, "Label.text in"="Ch2_ADC_Gain", "Master?"=w370, "Control Parameters [] in"=w354) -> ("Control Parameter"=w371:T16)  [unwired: 7 out]
      n146 = call "Get_Control_Parameter.vi"("Status/Errors in"=w353, "Label.text in"="Ch1_ADC_Gain", "Master?"=w365, "Control Parameters [] in"=w354) -> ("Control Parameter"=w368:T16)  [unwired: 7 out]
      n147 = call "Get_Control_Parameter.vi"("Status/Errors in"=w353, "Label.text in"="Ch2_ADC_Gain", "Master?"=w365, "Control Parameters [] in"=w354) -> ("Control Parameter"=w366:T16)  [unwired: 7 out]
      n148 = call "Get_Control_Parameter.vi"("Status/Errors in"=w353, "Label.text in"="Ch1_ADC_Offset", "Master?"=w360, "Control Parameters [] in"=w354) -> ("Control Parameter"=w363:T16)  [unwired: 7 out]
      n149 = call "Get_Control_Parameter.vi"("Status/Errors in"=w353, "Label.text in"="Ch2_ADC_Offset", "Master?"=w360, "Control Parameters [] in"=w354) -> ("Control Parameter"=w361:T16)  [unwired: 7 out]
      n150 = call "Get_Control_Parameter.vi"("Status/Errors in"=w353, "Label.text in"="Ch1_ADC_Offset", "Master?"=w355, "Control Parameters [] in"=w354) -> ("Control Parameter"=w358:T16)  [unwired: 7 out]
      n151 = call "Get_Control_Parameter.vi"("Status/Errors in"=w353, "Label.text in"="Ch2_ADC_Offset", "Master?"=w355, "Control Parameters [] in"=w354) -> ("Control Parameter"=w356:T16)  [unwired: 7 out]
      n152 = Unbundle By Name(w363) -> ("Min Real Value"=w346:dbl)
      n153 = Unbundle By Name(w361) -> ("Min Real Value"=w345:dbl)
      n154 = Unbundle By Name(w358) -> ("Min Real Value"=w347:dbl)
      n155 = Unbundle By Name(w356) -> ("Min Real Value"=w348:dbl)
      n156 = Unbundle By Name(w373) -> ("dReal/dByte"=w340:dbl)
      n157 = Unbundle By Name(w371) -> ("dReal/dByte"=w339:dbl)
      n158 = Unbundle By Name(w368) -> ("dReal/dByte"=w338:dbl)
      n159 = Unbundle By Name(w366) -> ("dReal/dByte"=w337:dbl)
      n160 = Multiply(x=w331, y=w340) -> (x*y=w333:dbl)
      n161 = Multiply(x=w331, y=w339) -> (x*y=w334:dbl)
      n162 = Multiply(x=w331, y=w338) -> (x*y=w335:dbl)
      n163 = Multiply(x=w331, y=w337) -> (x*y=w336:dbl)
      n164 = Add(x=w330, y=w346) -> (x+y=w341:dbl)
      n165 = Add(x=w330, y=w345) -> (x+y=w342:dbl)
      n166 = Add(x=w330, y=w347) -> (x+y=w343:dbl)
      n167 = Add(x=w330, y=w348) -> (x+y=w344:dbl)
      n168 = case shown="True" w332 {
        tunnel: [w382 w424] -> w375
        tunnel: w352 -> [_ w408]
        tunnel: w351 -> [_ w403]
        tunnel: w344 -> [_ w394]
        tunnel: w343 -> [_ w393]
        tunnel: w342 -> [_ w392]
        tunnel: w341 -> [_ w391]
        tunnel: w336 -> [_ w390]
        tunnel: w335 -> [_ w389]
        tunnel: w334 -> [_ w388]
        tunnel: w333 -> [_ w387]
        frame False {
          n169 = local read "timer"() -> (w377:u32)
          n170 = Tick Count (ms)() -> (millisecond timer value=w378:u32)
          n171 = Subtract(x=w378, y=w377) -> (x-y=w376:u32)
          n172 = case shown="True" "Start counting?" {
            tunnel: w378 -> [_ w384]
            frame False {
            }
            frame True {
              n173 = local write "Start counting?"(FALSE ("Start counting?")) -> ()
              "timer" <- w384
            }
          }
          n174 = Greater?(x=w376, y=u32 500) -> (0:→"Show traces?":bool)
          n175 = local read "Last trace"() -> (w382:dbl[][])
        }
        frame True {
          n176 = Delete From Array(array=w408, length=w403, index=0) -> (deleted portion=w402:u8[], array with subset deleted=w399:u8[])
          n177 = Delete From Array(array=w399, length=w403, index=0) -> (deleted portion=w401:u8[], array with subset deleted=w398:u8[])
          n178 = Delete From Array(array=w398, length=w403, index=24) -> (deleted portion=w400:u8[], array with subset deleted=w397:u8[])
          n179 = Delete From Array(array=w397, length=w403, index=24) -> (deleted portion=w395:u8[])  [unwired: 1 out]
          n180 = call "Byte_Array_To_12_Bit_Array.vi"("Byte-Array"=w402) -> ("12-Bit-Array"=w423:u16[])
          n181 = call "Byte_Array_To_12_Bit_Array.vi"("Byte-Array"=w401) -> ("12-Bit-Array"=w417:u16[])
          n182 = call "Byte_Array_To_12_Bit_Array.vi"("Byte-Array"=w400) -> ("12-Bit-Array"=w413:u16[])
          n183 = call "Byte_Array_To_12_Bit_Array.vi"("Byte-Array"=w395) -> ("12-Bit-Array"=w409:u16[])
          n184 = To Double Precision Float(number=w423) -> (double precision float=w422:dbl[])
          n185 = To Double Precision Float(number=w417) -> (double precision float=w419:dbl[])
          n186 = To Double Precision Float(number=w413) -> (double precision float=w415:dbl[])
          n187 = To Double Precision Float(number=w409) -> (double precision float=w411:dbl[])
          n188 = Multiply(x=w422, y=w387) -> (x*y=w421:dbl[])
          n189 = Multiply(x=w419, y=w388) -> (x*y=w418:dbl[])
          n190 = Multiply(x=w415, y=w389) -> (x*y=w414:dbl[])
          n191 = Multiply(x=w411, y=w390) -> (x*y=w410:dbl[])
          n192 = local write "Show traces?"(FALSE ("Show traces?")) -> ()
          n193 = local write "Start counting?"(TRUE ("Start counting?")) -> ()
          n194 = Add(x=w421, y=w391) -> (x+y=w420:dbl[])
          n195 = Add(x=w418, y=w392) -> (x+y=w416:dbl[])
          n196 = Add(x=w414, y=w393) -> (x+y=w412:dbl[])
          n197 = Add(x=w410, y=w394) -> (x+y=w396:dbl[])
          n198 = Build Array(w420, w416, w412, w396) -> (w424:dbl[][])
          "Last trace" <- w424
        }
      }
      n199 = Bundle(w333, w334, w335, w336) -> (w350:cluster{dbl, dbl, dbl, dbl})  [unwired: 1 out]
      n200 = Bundle(w341, w342, w343, w344) -> (w349:cluster{dbl, dbl, dbl, dbl})  [unwired: 1 out]
    }
  }
  n201 = Join Numbers(hi=w81, lo=w82) -> ((hi.lo)=w69:u16)
  n202 = Join Numbers(hi=w78, lo=w77) -> ((hi.lo)=w80:u16)
  n203 = Join Numbers(hi=w76, lo=w75) -> ((hi.lo)=w79:u16)
  n204 = Join Numbers(hi=w63, lo=w62) -> ((hi.lo)=w61:u16)
  n205 = Join Numbers(hi=w80, lo=w79) -> ((hi.lo)=w49:u32)
  n206 = Number To Boolean Array(number=w61) -> (Boolean array=w60:bool[])
  n207 = Number To Boolean Array(number=w30) -> (Boolean array=w28:bool[])
  n208 = Delete From Array(array=w60, index=9) -> (array with subset deleted=w58:bool[])  [unwired: 1 in, 1 out]
  n209 = Format Into String(format string="%02d-%02d-%04d, %02d:%02d:%02d, %d ns", initial string="", w71, w70, w69, w68, w67, w66, w49) -> (resulting string=w65:string, error out=w64:errorcluster)  [unwired: 1 in]
  n210 = Delete From Array(array=w58, index=15) -> (array with subset deleted=w27:bool[])  [unwired: 1 in, 1 out]
  n211 = Insert Into Array(array=w27, index=14, new element=w28) -> (w26:bool[])
  n212 = call "Check_For_Errors.vi"("Status/Errors in"=w47, "error in"=w64) -> ("Status/Errors out"=→"Status/Errors out":refnum<vi>)  [unwired: 9 out]
  n213 = Index Array(array=w26) -> (element #1=w25:bool, element #2=w24:bool, element #3=w23:bool, element #4=w22:bool, element #5=w21:bool, element #6=w20:bool, element #7=w19:bool, element #8=w18:bool, element #9=w17:bool, element #10=w16:bool, element #11=w15:bool, element #12=w14:bool, element #13=w13:bool, element #14=w12:bool, element #15=w11:bool, element #16=w10:bool, element #17=w9:bool, element #18=w8:bool)  [unwired: 18 in]
  n214 = case shown="1" w40 {
    tunnel: w43 -> [w426 w529 w583]
    tunnel: [w426 w518 w581] -> w41
    tunnel: w39 -> [_ w497 w580]
    tunnel: w36 -> [_ w476 w579]
    tunnel: [dbl[] [] w439 w540] -> w4
    frame Default {
    }
    frame 2 {
      # "Important!\n\nBefore calculating the statistics, the baseline is already substracted from the signal, therefore, the ADC offset is not substracted for the statistics Pulse height and integral. This is also the reason for the fact that the statistics on the front panel may dfiffer from what is actually seen from the traces."
      n215 = Index Array(array=w529, index #1=0 ("index"), index #2=1 ("index")) -> (element #1=w522:T15, element #2=w519:T15)
      n216 = Unbundle(w497) -> ("dReal/dByte"=w484:dbl, "dReal/dByte"=w483:dbl, "dReal/dByte"=w478:dbl, "dReal/dByte 2"=w477:dbl)
      n217 = Unbundle(w476) -> ("dReal/dByte"=w435:dbl, "dReal/dByte"=w436:dbl, "dReal/dByte"=w437:dbl, "dReal/dByte 2"=w438:dbl)
      n218 = Unbundle By Name(w522) -> ("Pulse height 1"=w517:i16, "Pulse height 2"=w516:i16, "Integral 1"=w515:i32, "Integral 2"=w514:i32, "Standard deviation 1"=w496:i16, "Standard deviation 2"=w495:i16, "Baseline 1"=w492:i16, "Baseline 2"=w491:i16)
      n219 = Unbundle By Name(w519) -> ("Pulse height 1"=w513:i16, "Pulse height 2"=w512:i16, "Integral 1"=w511:i32, "Integral 2"=w510:i32, "Standard deviation 1"=w494:i16, "Standard deviation 2"=w493:i16, "Baseline 1"=w490:i16, "Baseline 2"=w489:i16)
      n220 = To Double Precision Float(number=w517) -> (double precision float=w502:dbl)
      n221 = To Double Precision Float(number=w516) -> (double precision float=w503:dbl)
      n222 = To Double Precision Float(number=w515) -> (double precision float=w504:dbl)
      n223 = To Double Precision Float(number=w514) -> (double precision float=w505:dbl)
      n224 = To Double Precision Float(number=w496) -> (double precision float=w485:dbl)
      n225 = To Double Precision Float(number=w495) -> (double precision float=w486:dbl)
      n226 = To Double Precision Float(number=w492) -> (double precision float=w487:dbl)
      n227 = To Double Precision Float(number=w491) -> (double precision float=w488:dbl)
      n228 = To Double Precision Float(number=w513) -> (double precision float=w506:dbl)
      n229 = To Double Precision Float(number=w512) -> (double precision float=w507:dbl)
      n230 = To Double Precision Float(number=w511) -> (double precision float=w508:dbl)
      n231 = To Double Precision Float(number=w510) -> (double precision float=w509:dbl)
      n232 = To Double Precision Float(number=w494) -> (double precision float=w482:dbl)
      n233 = To Double Precision Float(number=w493) -> (double precision float=w481:dbl)
      n234 = To Double Precision Float(number=w490) -> (double precision float=w480:dbl)
      n235 = To Double Precision Float(number=w489) -> (double precision float=w479:dbl)
      n236 = Multiply(x=w504, y=w484) -> (x*y=w501:dbl)
      n237 = Multiply(x=w502, y=w484) -> (x*y=w465:dbl)
      n238 = Multiply(x=w503, y=w483) -> (x*y=w466:dbl)
      n239 = Multiply(x=w505, y=w483) -> (x*y=w500:dbl)
      n240 = Multiply(x=w485, y=w484) -> (x*y=w471:dbl)
      n241 = Multiply(x=w486, y=w483) -> (x*y=w440:dbl)
      n242 = Multiply(x=w487, y=w484) -> (x*y=w434:dbl)
      n243 = Multiply(x=w488, y=w483) -> (x*y=w433:dbl)
      n244 = Multiply(x=w506, y=w478) -> (x*y=w464:dbl)
      n245 = Multiply(x=w507, y=w477) -> (x*y=w463:dbl)
      n246 = Multiply(x=w508, y=w478) -> (x*y=w499:dbl)
      n247 = Multiply(x=w509, y=w477) -> (x*y=w498:dbl)
      n248 = Multiply(x=w482, y=w478) -> (x*y=w470:dbl)
      n249 = Multiply(x=w481, y=w477) -> (x*y=w469:dbl)
      n250 = Multiply(x=w480, y=w478) -> (x*y=w432:dbl)
      n251 = Multiply(x=w479, y=w477) -> (x*y=w431:dbl)
      n252 = Add(x=w434, y=w435) -> (x+y=w430:dbl)
      n253 = Add(x=w433, y=w436) -> (x+y=w429:dbl)
      n254 = Add(x=w432, y=w437) -> (x+y=w428:dbl)
      n255 = Add(x=w431, y=w438) -> (x+y=w427:dbl)
      n256 = Multiply(x=w501, y=2.5) -> (x*y=w467:dbl)
      n257 = Multiply(x=w500, y=2.5) -> (x*y=w468:dbl)
      n258 = Multiply(x=w499, y=2.5) -> (x*y=w462:dbl)
      n259 = Multiply(x=w498, y=2.5) -> (x*y=w461:dbl)
      n260 = Build Array(w430, w429, w428, w427) -> (w439:dbl[])
      n261 = Add(x=w434, y=w435) -> (x+y=w475:dbl)
      n262 = Add(x=w433, y=w436) -> (x+y=w474:dbl)
      n263 = Add(x=w432, y=w437) -> (x+y=w473:dbl)
      n264 = Add(x=w431, y=w438) -> (x+y=w472:dbl)
      n265 = To Word Integer(number=w465) -> (16bit integer=w449:i16)
      n266 = To Word Integer(number=w466) -> (16bit integer=w450:i16)
      n267 = To Long Integer(number=w467) -> (32bit integer=w451:i32)
      n268 = To Long Integer(number=w468) -> (32bit integer=w452:i32)
      n269 = To Word Integer(number=w471) -> (16bit integer=w447:i16)
      n270 = To Word Integer(number=w440) -> (16bit integer=w446:i16)
      n271 = To Word Integer(number=w475) -> (16bit integer=w453:i16)
      n272 = To Word Integer(number=w474) -> (16bit integer=w454:i16)
      n273 = To Word Integer(number=w464) -> (16bit integer=w455:i16)
      n274 = To Word Integer(number=w463) -> (16bit integer=w456:i16)
      n275 = To Long Integer(number=w462) -> (32bit integer=w457:i32)
      n276 = To Long Integer(number=w461) -> (32bit integer=w458:i32)
      n277 = To Word Integer(number=w470) -> (16bit integer=w444:i16)
      n278 = To Word Integer(number=w469) -> (16bit integer=w442:i16)
      n279 = To Word Integer(number=w473) -> (16bit integer=w459:i16)
      n280 = To Word Integer(number=w472) -> (16bit integer=w460:i16)
      n281 = Absolute Value(x=w444) -> (abs(x)=w443:i16)
      n282 = Absolute Value(x=w442) -> (abs(x)=w441:i16)
      n283 = Absolute Value(x=w447) -> (abs(x)=w448:i16)
      n284 = Absolute Value(x=w446) -> (abs(x)=w445:i16)
      n285 = Bundle By Name(cluster=w522, "Pulse height 1"=w449, "Pulse height 2"=w450, "Integral 1"=w451, "Integral 2"=w452, "Standard deviation 1"=w448, "Standard deviation 2"=w445, "Baseline 1"=w453, "Baseline 2"=w454) -> (w521:T15)
      n286 = Bundle By Name(cluster=w519, "Pulse height 1"=w455, "Pulse height 2"=w456, "Integral 1"=w457, "Integral 2"=w458, "Standard deviation 1"=w443, "Standard deviation 2"=w441, "Baseline 1"=w459, "Baseline 2"=w460) -> (w520:T15)
      n287 = Build Array(w521, w520) -> (w518:T15[])
    }
    frame 1 {
      n288 = Index Array(array=w583, index=0) -> (element=w554:T15)
      n289 = Unbundle(w580) -> ("dReal/dByte"=w555:dbl, "dReal/dByte"=w556:dbl)  [unwired: 2 out]
      n290 = Unbundle(w579) -> ("dReal/dByte"=w535:dbl, "dReal/dByte"=w534:dbl)  [unwired: 2 out]
      n291 = Unbundle By Name(w554) -> ("Pulse height 1"=w576:i16, "Pulse height 2"=w575:i16, "Integral 1"=w574:i32, "Integral 2"=w573:i32, "Standard deviation 1"=w566:i16, "Standard deviation 2"=w565:i16, "Baseline 1"=w564:i16, "Baseline 2"=w563:i16)
      n292 = To Double Precision Float(number=w576) -> (double precision float=w569:dbl)
      n293 = To Double Precision Float(number=w575) -> (double precision float=w570:dbl)
      n294 = To Double Precision Float(number=w574) -> (double precision float=w571:dbl)
      n295 = To Double Precision Float(number=w573) -> (double precision float=w572:dbl)
      n296 = To Double Precision Float(number=w566) -> (double precision float=w559:dbl)
      n297 = To Double Precision Float(number=w565) -> (double precision float=w560:dbl)
      n298 = To Double Precision Float(number=w564) -> (double precision float=w561:dbl)
      n299 = To Double Precision Float(number=w563) -> (double precision float=w562:dbl)
      n300 = Multiply(x=w571, y=w555) -> (x*y=w568:dbl)
      n301 = Multiply(x=w569, y=w555) -> (x*y=w530:dbl)
      n302 = Multiply(x=w570, y=w556) -> (x*y=w531:dbl)
      n303 = Multiply(x=w572, y=w556) -> (x*y=w567:dbl)
      n304 = Multiply(x=w559, y=w555) -> (x*y=w552:dbl)
      n305 = Multiply(x=w560, y=w556) -> (x*y=w551:dbl)
      n306 = Multiply(x=w561, y=w555) -> (x*y=w537:dbl)
      n307 = Multiply(x=w562, y=w556) -> (x*y=w536:dbl)
      n308 = Add(x=w537, y=w535) -> (x+y=w538:dbl)
      n309 = Add(x=w536, y=w534) -> (x+y=w539:dbl)
      n310 = Multiply(x=w568, y=2.5) -> (x*y=w532:dbl)
      n311 = Multiply(x=w567, y=2.5) -> (x*y=w533:dbl)
      n312 = Build Array(w538, w539) -> (w540:dbl[])
      n313 = Add(x=w537, y=w535) -> (x+y=w558:dbl)
      n314 = Add(x=w536, y=w534) -> (x+y=w557:dbl)
      n315 = To Word Integer(number=w530) -> (16bit integer=w549:i16)
      n316 = To Word Integer(number=w531) -> (16bit integer=w548:i16)
      n317 = To Long Integer(number=w532) -> (32bit integer=w550:i32)
      n318 = To Long Integer(number=w533) -> (32bit integer=w541:i32)
      n319 = To Word Integer(number=w552) -> (16bit integer=w545:i16)
      n320 = To Word Integer(number=w551) -> (16bit integer=w543:i16)
      n321 = To Word Integer(number=w558) -> (16bit integer=w547:i16)
      n322 = To Word Integer(number=w557) -> (16bit integer=w546:i16)
      n323 = Absolute Value(x=w545) -> (abs(x)=w544:i16)
      n324 = Absolute Value(x=w543) -> (abs(x)=w542:i16)
      n325 = Bundle By Name(cluster=w554, "Pulse height 1"=w549, "Pulse height 2"=w548, "Integral 1"=w550, "Integral 2"=w541, "Standard deviation 1"=w544, "Standard deviation 2"=w542, "Baseline 1"=w547, "Baseline 2"=w546) -> (w553:T15)
      n326 = Build Array(w553) -> (w581:T15[])
    }
  }
  "Event statistics" <- w41
  n327 = Insert Into Array(array=w6, index (col)=0 ("disabled index (col)"), new element=w4) -> (w7:dbl[][])  [unwired: 1 in]
  n328 = Bundle By Name(cluster=T17 {"Det_Numb"=0, "GPS_Timestamp"="", "Trigger_Pattern"={"Master ch. 1 lower threshold"=FALSE, "Master ch. 1 higher threshold"=FALSE, "Master ch. 2 lower threshold"=FALSE, "Master ch. 2 higher threshold"=FALSE, "Slave ch. 1 lower threshold"=FALSE, "Slave ch. 1 higher threshold"=FALSE, "Slave ch. 2 lower threshold"=FALSE, "Slave ch. 2 higher threshold"=FALSE, "External trigger"=FALSE, "Slave present?"=FALSE, "Ch. 1 low comparator master"=FALSE, "Ch. 1 high comparator master"=FALSE, "Ch. 2 low comparator master"=FALSE, "Ch. 2 high comparator master"=FALSE, "Ch. 1 low comparator slave"=FALSE, "Ch. 1 high comparator slave"=FALSE, "Ch. 2 low comparator slave"=FALSE, "Ch. 2 high comparator slave"=FALSE}, "Traces"=[], "MAS_Status_Events"=FALSE, "MAS_Vers_Numb"="", "SLV_Status_Events"=FALSE, "SLV_Vers_Numb"="", "DBase_connected?"=FALSE, "MAS_GPS_Long"=0.0, "MAS_GPS_Lat"=0.0, "MAS_GPS_Alt"=0.0, "Hardware"=enum."None"} ("GEN_Page_Events"), "GPS_Timestamp"=w65, "Trigger_Pattern.Master ch. 1 lower threshold"=w25, "Trigger_Pattern.Master ch. 1 higher threshold"=w24, "Trigger_Pattern.Master ch. 2 lower threshold"=w23, "Trigger_Pattern.Master ch. 2 higher threshold"=w22, "Trigger_Pattern.Slave ch. 1 lower threshold"=w21, "Trigger_Pattern.Slave ch. 1 higher threshold"=w20, "Trigger_Pattern.Slave ch. 2 lower threshold"=w19, "Trigger_Pattern.Slave ch. 2 higher threshold"=w18, "Trigger_Pattern.External trigger"=w17, "Trigger_Pattern.Slave present?"=w16, "Trigger_Pattern.Ch. 1 low comparator master"=w15, "Trigger_Pattern.Ch. 1 high comparator master"=w14, "Trigger_Pattern.Ch. 2 low comparator master"=w13, "Trigger_Pattern.Ch. 2 high comparator master"=w12, "Trigger_Pattern.Ch. 1 low comparator slave"=w11, "Trigger_Pattern.Ch. 1 high comparator slave"=w10, "Trigger_Pattern.Ch. 2 low comparator slave"=w9, "Trigger_Pattern.Ch. 2 high comparator slave"=w8, "Traces"=w7) -> (→"Event cluster":T17)
  "Main parameters out" <- "Main parameters in"
